vi "仓库关联远程.vi"(4 "密码":string, 6 "用户名":string, 8 "error in":errorcluster caption="错误输入（无错误）", 10 "远程仓库":string, 11 "仓库路径":path) -> (0 "error out":errorcluster caption="错误输出", 1 "standard error":string caption="标准错误", 2 "standard output":string caption="标准输出", 3 "仓库路径":path)   [LabVIEW 2018]
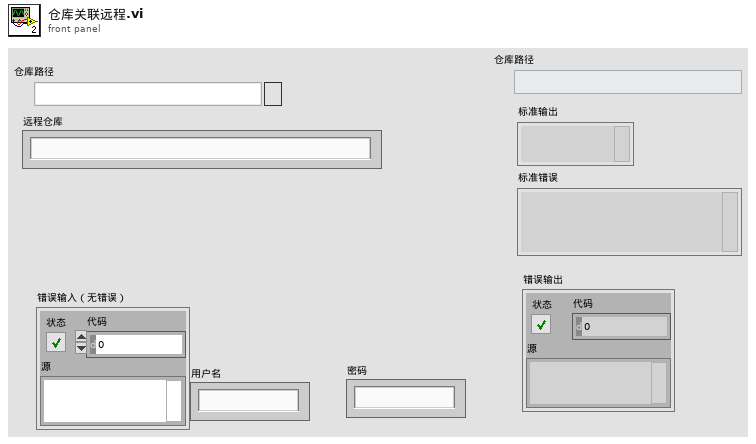
[diagram p1: front panel]
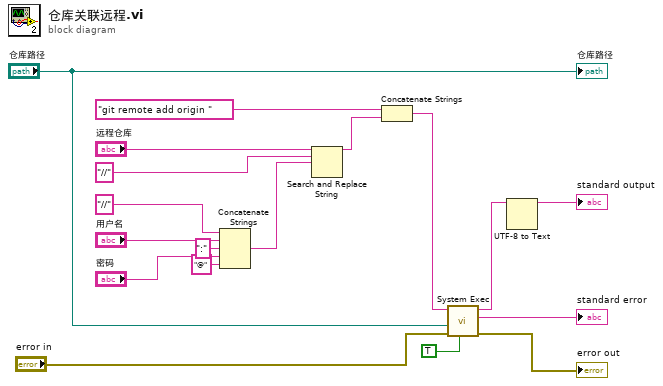
[diagram p0: block diagram]
diagram:
  n1 = Concatenate Strings("//" ("字符串"), "用户名", ":" ("字符串"), "密码", "@" ("字符串")) -> (w4:string)
  n2 = Search and Replace String(input string="远程仓库", search string="//" ("搜索字符串"), replace string=w4) -> (result string=w3:string)  [unwired: 5 in, 3 out]
  n3 = Concatenate Strings("git remote add origin " ("command line"), w3) -> (w11:string)
  n4 = call <vilib>:"System Exec.vi"("run minimized? (F)"=TRUE, "error in (no error)"="error in", "working directory"="仓库路径", "command line"=w11) -> ("error out"=→"error out":errorcluster, "standard error"=→"standard error":string, "standard output"=w17:string)  [unwired: 4 in, 1 out]
  n5 = UTF-8 to Text ("UTF-8至文本转换")(11:w17) -> (3:→"standard output":string)  [unwired: 2 in, 1 out]
  "仓库路径" <- "仓库路径"
